vi "Create Differential Plot Single Channel.vi"(6 "Upper Limit":dbl, 8 "Error In":errorcluster, 9 "Lower Limit":dbl, 10 "Differential Value":dbl format="%#_13g", 11 "Dev1 Ch3":dynamicdata(waveform)) -> (0 "Error Out":errorcluster, 3 "Array":cluster{"Array":dbl[], "Array":dbl[]}[](array[cluster]))   [LabVIEW 2017]
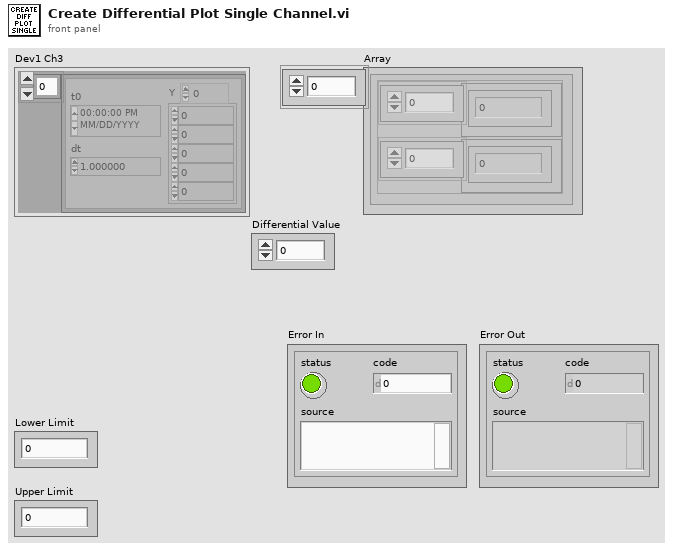
[diagram p1: front panel]
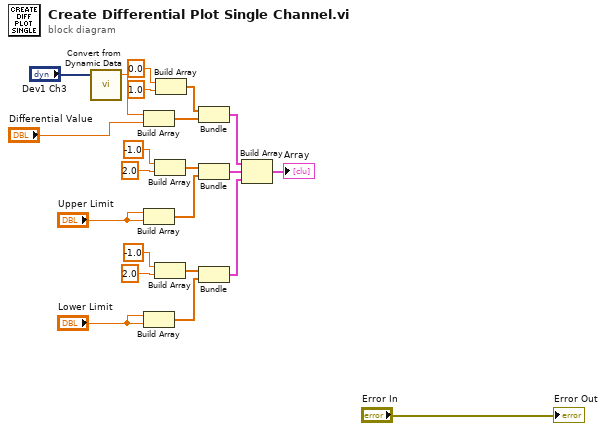
[diagram p0: block diagram]
diagram:
  n1 = call "Convert from Dynamic Data"("Dynamic Data Type"="Dev1 Ch3") -> ("Scalar"=w4:dbl)  [unwired: 3 in]
  n2 = Build Array(w4, "Differential Value") -> (w7:dbl[])
  n3 = Build Array("Upper Limit", "Upper Limit") -> (w16:dbl[])
  n4 = Build Array("Lower Limit", "Lower Limit") -> (w18:dbl[])
  n5 = Build Array(-1.0 ("element"), 2.0 ("element")) -> (w14:dbl[])
  n6 = Build Array(-1.0 ("element"), 2.0 ("element")) -> (w17:dbl[])
  n7 = Build Array(0.0 ("element"), 1.0 ("element")) -> (w8:dbl[])
  n8 = Bundle(w8, w7) -> (w11:cluster{dbl[], dbl[]})  [unwired: 1 in]
  n9 = Bundle(w14, w16) -> (w12:cluster{dbl[], dbl[]})  [unwired: 1 in]
  n10 = Bundle(w17, w18) -> (w22:cluster{dbl[], dbl[]})  [unwired: 1 in]
  n11 = Build Array(w11, w12, w22) -> (→"Array":cluster{dbl[], dbl[]}[])
  "Error Out" <- "Error In"
